vi "NISE.remote.Read Dev.Commands.vi"(8 "error in (no error)":errorcluster, 11 "SLSC Remote in":refnum<class "SLSC Interface.lvclass">) -> (0 "error out":errorcluster, 2 "Dev.Commands":refnum<k21>[](array[refnum]), 3 "SLSC Remote out":refnum<class "SLSC Interface.lvclass">)   [LabVIEW 2016, in "SLSC Interface.lvclass"]
uses:
  SLSC Interface Class/SLSC Interface.lvclass
  <vilib>/NI/JSON Support for LabVIEW/JSON Value/JSON Value.lvclass
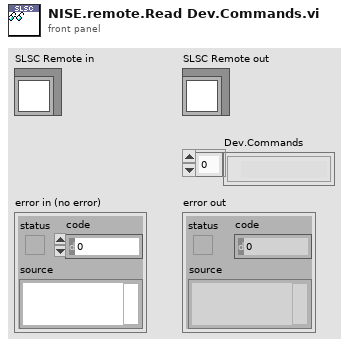
[diagram p1: front panel]
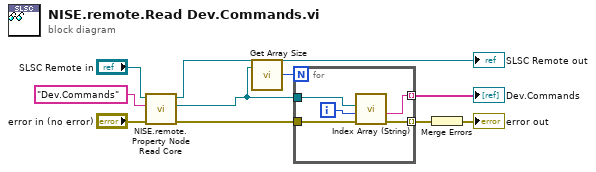
[diagram p0: block diagram]
diagram:
  n1 = call "NISE.remote.Property Node Read Core.vi"("error in (no error)"="error in (no error)", "property"="Dev.Commands", "SLSC Remote in"="SLSC Remote in") -> ("error out"=w4:errorcluster, "JSON Value out"=w1:refnum<class "JSON Value.lvclass">, "SLSC Remote out"=→"SLSC Remote out":refnum<class "SLSC Interface.lvclass">)  [unwired: 6 in]
  n2 = call <vilib>:"Get Array Size.vi"("JSON Value in"=w1) -> ("size(s)"=w6:i32)  [unwired: 1 in, 1 out]
  n3 = for {
    N: w6 -> [_]
    tunnel: w1 -> [w15]
    tunnel: [w13] -> w5 mode=indexing
    tunnel: w4 -> [w12]
    tunnel: [w11] -> w3 mode=indexing
    i -> [w14]
    n4 = call <vilib>:"Index Array (String).vi"("error in (no error)"=w12, "index"=w14, "JSON Value in"=w15) -> ("error out"=w11:errorcluster, "String"=w13:string)  [unwired: 7 in]
  }
  "Dev.Commands" <- w5
  n5 = Merge Errors(w3) -> (→"error out":errorcluster)
